vi "Read clock id.vi"(8 "error in (no error)":errorcluster, 11 "Cond in":refnum<class "Cond.lvclass">) -> (0 "error out":errorcluster, 2 "lv_clockid_t":T1=enum."Monotonic", 3 "Cond out":refnum<class "Cond.lvclass">)   [LabVIEW 2013, in "Linux RT IPC.lvlib" / "POSIX Threads.lvlib" / "Cond.lvclass"]
uses:
  Cond.lvclass
  <vilib>/NI/NI Linux RT Utilities/Controls/Public/C Enums/clockid_t.ctl
  Cond.lvclass/Cond.ctl
  <vilib>/NI/NI Linux RT Utilities/Linux RT Utilities.lvlib
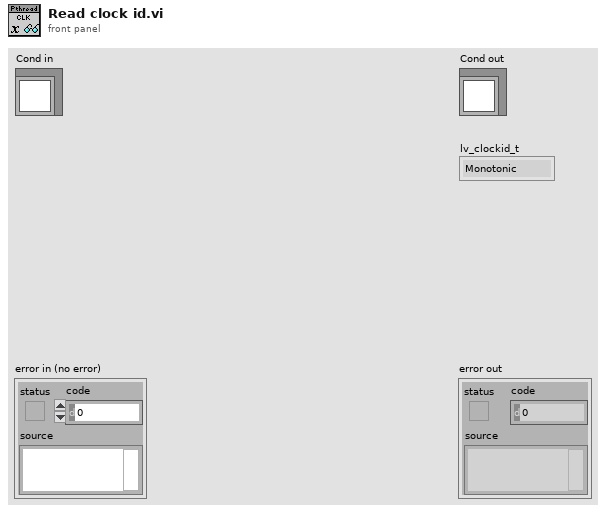
[diagram p1: front panel]
types:
  T1 = typedef "Linux RT Utilities.lvlib/clockid_t.ctl" = enum16{"Realtime", "Monotonic"}
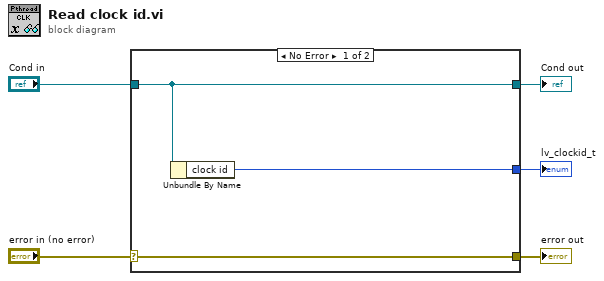
[diagram p0: block diagram]
diagram:
  n1 = case shown="No Error" "error in (no error)" {
    selector: "error in (no error)" -> [w8 w9]
    tunnel: [w8 w9] -> w4
    tunnel: [w7 w10] -> w2
    tunnel: "Cond in" -> [w7 w10]
    tunnel: [w6 _] -> w1
    frame No Error {
      n2 = Unbundle By Name(w7) -> ("clock id"=w6:T1)
    }
    frame Error {
    }
  }
  "error out" <- w4
  "Cond out" <- w2
  "lv_clockid_t" <- w1
